vi "FindInstruments.vi"(8 "error in (no error)":errorcluster, 11 "Hamamatsu_Camera in":refnum<class "Hamamatsu_Camera.lvclass">) -> (0 "error out":errorcluster, 3 "Hamamatsu_Camera out":refnum<class "Hamamatsu_Camera.lvclass">)   [LabVIEW 2023, in "Hamamatsu_Camera.lvlib" / "Hamamatsu_Camera.lvclass"]
uses:
  Hamamatsu_Camera.lvclass
  C:/Program Files/National Instruments/LabVIEW 2023/vi.lib/ActorFramework/Actor/Actor.lvclass
  <vilib>/ActorFramework/Actor/Actor.lvclass/Actor.ctl
  Hamamatsu_Camera.lvclass/Hamamatsu_Camera.ctl
  Interfaces/InitDeinitInterface/InitDeinitComm Messages/FoundInstruments Msg/FoundInstruments Msg.lvclass/FoundInstruments Msg.ctl
  <vilib>/ActorFramework/Message Enqueuer/Message Enqueuer.lvclass/Message Enqueuer.ctl
  <vilib>/ActorFramework/Message Enqueuer/Enqueue.vi
  Interfaces/InitDeinitInterface/InitDeinitComm Messages/FoundInstruments Msg/FoundInstruments Msg.lvclass
  C:/Program Files/National Instruments/LabVIEW 2023/vi.lib/ActorFramework/Message/Message.lvclass
  <vilib>/ActorFramework/Message Priority Queue/Priority Enqueue.vi
  <vilib>/ActorFramework/Actor/Actor.lvclass
panel:
  in  "Instruments Found":T1
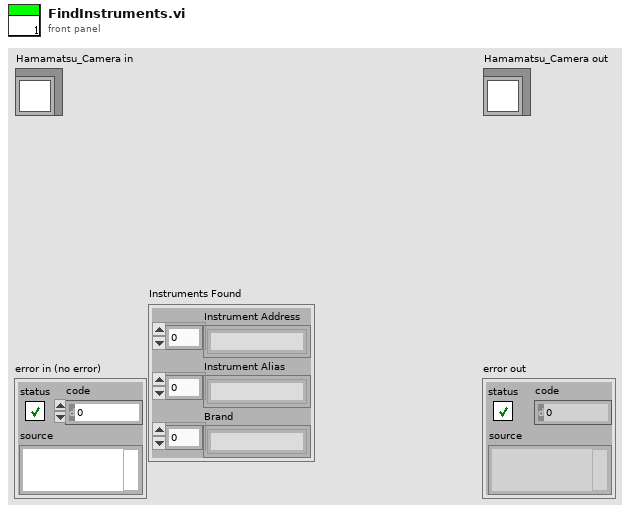
[diagram p1: front panel]
types:
  T1 = cluster{"Instrument Address":string[], "Instrument Alias":string[], "Brand":string[]}
  T2 = cluster{"Model":string, "Camera ID":string, "Firmware":string}[]
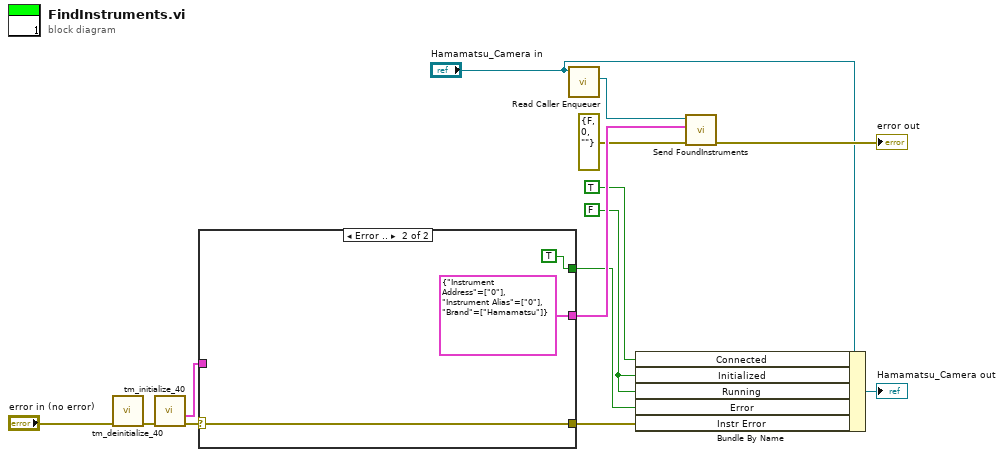
[diagram p0: block diagram]
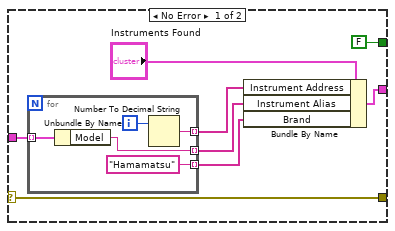
[diagram p2: hidden frame]
diagram:
  w5 = FALSE ("InstrumentData.CurrentState.Running")
  n1 = call "tm_deinitialize_40.vi"("error in (no error)"="error in (no error)") -> ("error out"=w9:errorcluster)  [unwired: 10 in]
  n2 = call "tm_initialize_40.vi"("error in (no error)"=w9) -> ("error out"=w8:errorcluster, "Camera Details Array"=w12:T2)  [unwired: 7 in, 2 out]
  n3 = case shown="Error .." w8 {
    selector: w8 -> [w15 w28]
    tunnel: w12 -> [w22 _]
    tunnel: [w19 T1 {"Instrument Address"=["0"], "Instrument Alias"=["0"], "Brand"=["Hamamatsu"]} ("Instruments Found")] -> w11
    tunnel: [FALSE ("InstrumentData.CurrentState.Error") TRUE ("InstrumentData.CurrentState.Error")] -> w4
    tunnel: [w15 w28] -> w3
    frame No Error {
      n4 = for {
        tunnel: w22 -> [w27] mode=indexing
        tunnel: [w26] -> w20 mode=indexing
        tunnel: [w24] -> w18 mode=indexing
        tunnel: ["Hamamatsu"] -> w17 mode=indexing
        i -> [w25]
        n5 = Unbundle By Name(w27) -> ("Model"=w26:string)
        n6 = Number To Decimal String(number=w25) -> (decimal integer string=w24:string)  [unwired: 1 in]
      }
      n7 = Bundle By Name(cluster="Instruments Found", "Instrument Address"=w18, "Instrument Alias"=w20, "Brand"=w17) -> (w19:T1)
    }
    frame Error {
    }
  }
  n8 = call <vilib>:"Read Caller Enqueuer.vi"("Actor"="Hamamatsu_Camera in") -> ("Caller Enqueuer"=w14:refnum<class "Message Enqueuer.lvclass">)  [unwired: 10 in]
  n9 = Bundle By Name(cluster="Hamamatsu_Camera in", "Connected"=TRUE ("InstrumentData.CurrentState.Connected"), "Initialized"=w5, "Running"=w5, "Error"=w4, "Instr Error"=w3) -> (→"Hamamatsu_Camera out":refnum<class "Hamamatsu_Camera.lvclass">)
  n10 = call "Send FoundInstruments.vi"("error in (no error)"=errorcluster {"status"=FALSE, "code"=0, "source"=""}, "Instruments Found"=w11, "Message Enqueuer"=w14) -> ("error out"=→"error out":errorcluster)  [unwired: 7 in, 1 out]
